vi "CH_LM Action Trend StartStop.vi"(0 "Meter Index":i32, 2 "Start/Stop (start)":bool=TRUE, 3 "File Name (\"\")":string, 5 "error in (no error)":errorcluster, 7 "Timeout / ms (3000)":i32=3000, 9 "Lock Timeout / ms (1000)":i32=1000) -> (11 "Lock timed out":bool, 14 "Meter Index":i32, 19 "error out":errorcluster)   [LabVIEW 2012, in "CH_LM.lvlib"]
doc: "This command will initiate/restart or terminate a trend cycle.\n\n<B>Note:</B> This command will be ignored if trend display mode is not active."
uses:
  CH_LM.lvlib
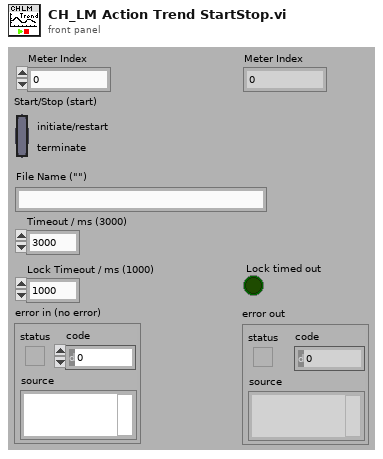
[diagram p1: front panel]
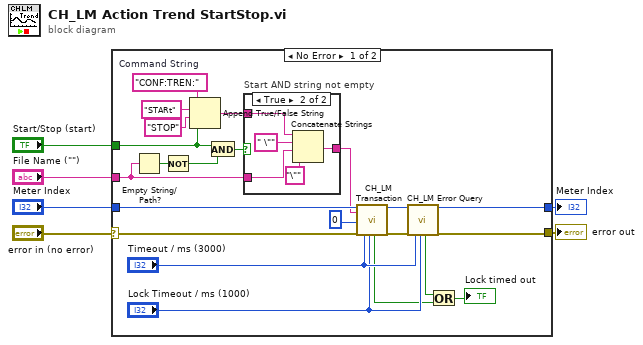
[diagram p0: block diagram]
diagram:
  n1 = case shown="No Error" "error in (no error)" {
    selector: "error in (no error)" -> [w28 w36]
    tunnel: [w26 w36] -> w6
    tunnel: "Meter Index" -> [w27 w35]
    tunnel: [w25 w35] -> w3
    tunnel: "Start/Stop (start)" -> [w9 _]
    tunnel: "File Name (\"\")" -> [w11 _]
    frame No Error {
      w17 = "CONF:TREN:"  # Command String
      n2 = Empty String/Path?(string/path=w11) -> (empty?=w10:bool)
      n3 = Not(x=w10) -> (.not. x?=w7:bool)
      n4 = Append True/False String(1:w9, 2:"STOP" ("false string"), 3:"STARt" ("true string"), 4:w17) -> (0:w13:string)
      n5 = And(x=w9, y=w7) -> (x .and. y?=w8:bool)
      n6 = case "Start AND string not empty" shown="True" w8 {
        tunnel: w13 -> [w29 w34]
        tunnel: [w29 w33] -> w12
        tunnel: w11 -> [_ w31]
        frame False {
        }
        frame True {
          n7 = Concatenate Strings(w34, " \"", w31, "\"" ("string")) -> (w33:string)
        }
      }
      n8 = call "CH_LM Transaction.vi"("Meter Index"=w27, "Command String"=w12, "NofStrings (-1:all)"=0 ("t"), "error in (no error)"=w28, "Timeout / ms (3000)"="Timeout / ms (3000)", "Lock Timeout / ms (1000)"="Lock Timeout / ms (1000)") -> ("Lock timed out"=w19:bool, "Meter Index"=w22:i32, "error out"=w21:errorcluster)  [unwired: 11 out]
      n9 = call "CH_LM Error Query.vi"("Meter Index"=w22, "error in (no error)"=w21, "Timeout / ms (3000)"="Timeout / ms (3000)", "Lock Timeout / ms (1000)"="Lock Timeout / ms (1000)") -> ("Lock timed out"=w20:bool, "Meter Index"=w25:i32, "error out"=w26:errorcluster)  [unwired: 13 out]
      n10 = Or(x=w20, y=w19) -> (x .or. y?=→"Lock timed out":bool)
    }
    frame Error {
    }
  }
  "error out" <- w6
  "Meter Index" <- w3
